vi "Autonomous Independent.vi"   [LabVIEW 2013]
doc: "This VI is called when autonomous begins, and will automatically be terminated when autonomous ends. You can carry out timed or sensor driven robot movement independently without needing to return to the caller."
uses:
  Gyro/Gyro Global.vi
  Robot Global Data.vi
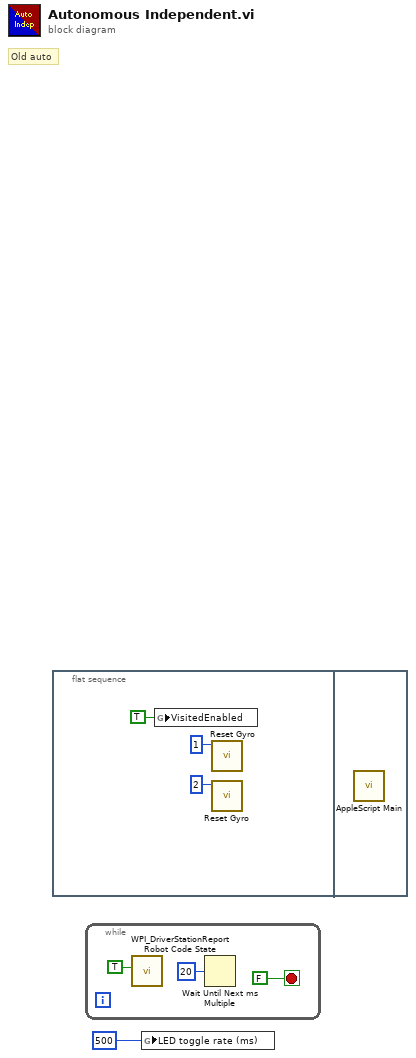
[diagram p0: block diagram]
diagram:
  # "Old auto"
  n1 = flat-sequence {
    frame #0 {
      n2 = global write "Gyro Global.vi" "VisitedEnabled"(TRUE ("VisitedEnabled")) -> ()
      n3 = call "Reset Gyro.vi"("Gyro ID (1 or 2)"=1) -> ()  [unwired: 11 in]
      n4 = call "Reset Gyro.vi"("Gyro ID (1 or 2)"=2) -> ()  [unwired: 11 in]
    }
    frame #1 {
      n5 = call "AppleScript Main.vi"() -> ()  [unwired: 12 in]
    }
  }
  n6 = while {
    stop <- FALSE stop-if-true
    n7 = call <vilib>:"WPI_DriverStationReport Robot Code State.vi"("Autonomous"=TRUE) -> ()  [unwired: 10 in, 1 out]
    n8 = Wait Until Next ms Multiple(millisecond multiple=u32 20 ("milliseconds to wait")) -> ()  [unwired: 1 out]
  }
  n9 = global write "Robot Global Data.vi" "LED toggle rate (ms)"(u32 500 ("LED ms toggle rate")) -> ()
